vi "AO SCTR Engine.vi"(0 "Unique Notifier Name":string, 11 "AO PFI Lines":string[](array[string])) -> ()   [LabVIEW 2016]
uses:
  AO SCTR Type Defs/AO SCTR Notifier Type.ctl
  AO SCTR Type Defs/AO SCTR Actions.ctl
  <vilib>/DAQmx/write.llb/DAQmx Write (Analog DBL 1Chan 1Samp).vi
  <vilib>/Analysis/1siggen.llb/Ramp Pattern by Samples.vi
  <vilib>/DAQmx/write.llb/DAQmx Write (Analog 1D DBL 1Chan NSamp).vi
  <vilib>/DAQmx/create/channels.llb/DAQmx Create Channel (AO-Voltage-Basic).vi
  <vilib>/DAQmx/miscellaneous.llb/DAQmx Fill In Error Info.vi
  <vilib>/DAQmx/configure/timing.llb/DAQmx Timing (Sample Clock).vi
  <resource>/objmgr/daqmx.rc
  <vilib>/Analysis/NI_AALBase.lvlib
panel:
  out "Running":bool
  in  "Load":bool
  in  "Save":bool
  in  "Quit":bool
  in  "Waveform Settings":T1={"Actions"=enum."Offset", "Mirror Offset (V)"=-0.61, "Mirror Amplititude (V)"=0.524, "Samples Per Channel"=2280, "Start Delay (ms)"=20.0, "Running?"=FALSE} {"Mirror Amplititude (V)" format="%#_13g"; "Mirror Offset (V)" format="%#_13g"; "Start Delay (ms)" format="%#_13g"}
  out "Waveform Graph":dbl[](graph)
  out "Actual Sample Rate":dbl=10000.0 format="%0.2f"
  # "AO Line Example: Dev1/ao1\nPFI Line Example: /Dev1/PFI0"
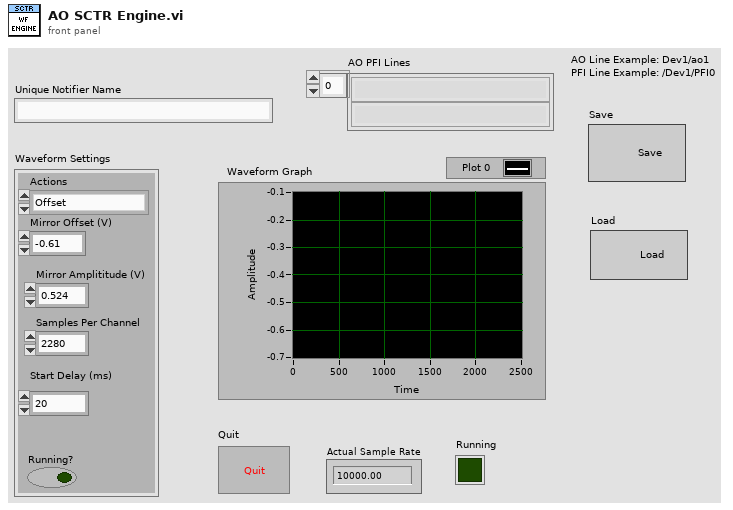
[diagram p1: front panel]
types:
  T1 = typedef "AO SCTR Notifier Type.ctl" = cluster{"Actions":T2, "Mirror Offset (V)":dbl, "Mirror Amplititude (V)":dbl, "Samples Per Channel":i32, "Start Delay (ms)":dbl, "Running?":bool}
  T2 = typedef "AO SCTR Actions.ctl" = enum16{"Offset", "Run", "Quit"}
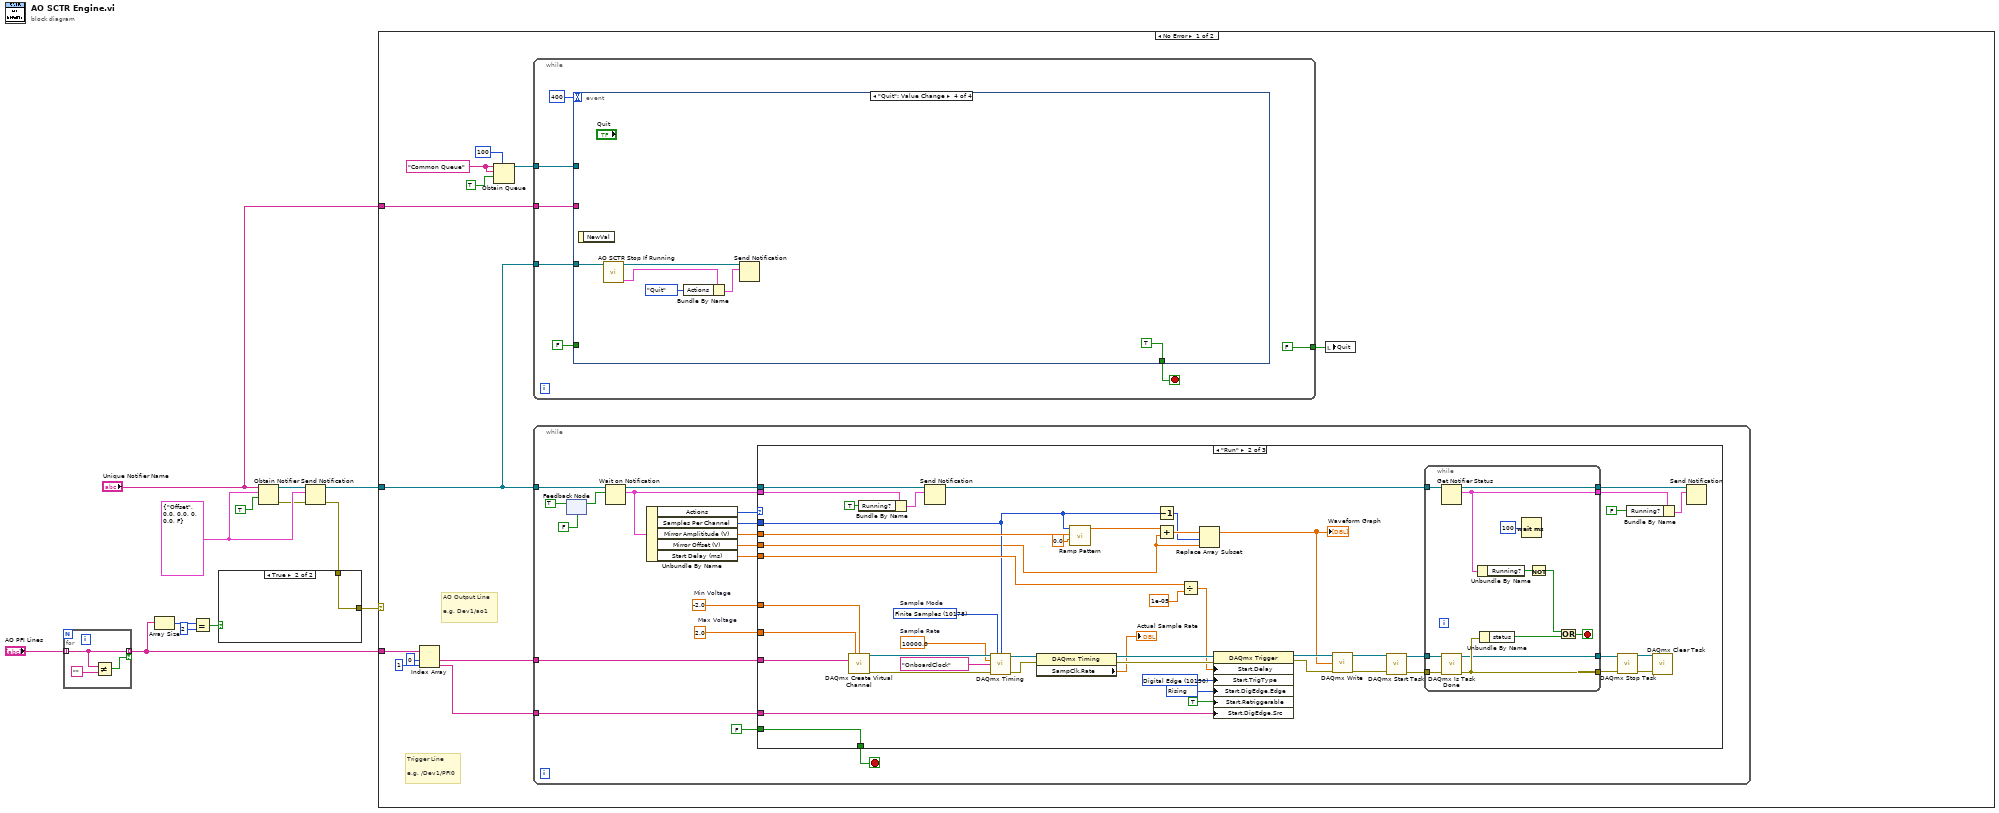
[diagram p0: block diagram]
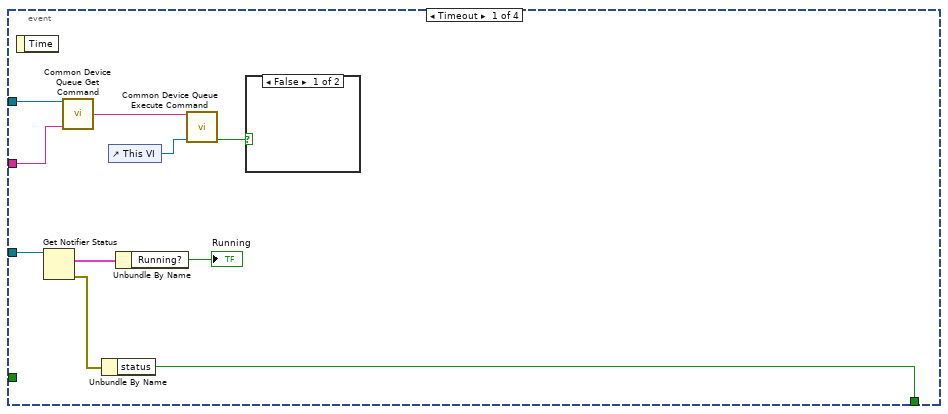
[diagram p2: hidden frame]
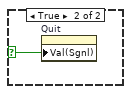
[diagram p3: hidden frame]
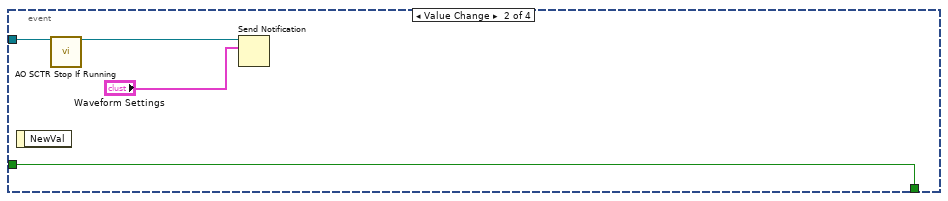
[diagram p4: hidden frame]
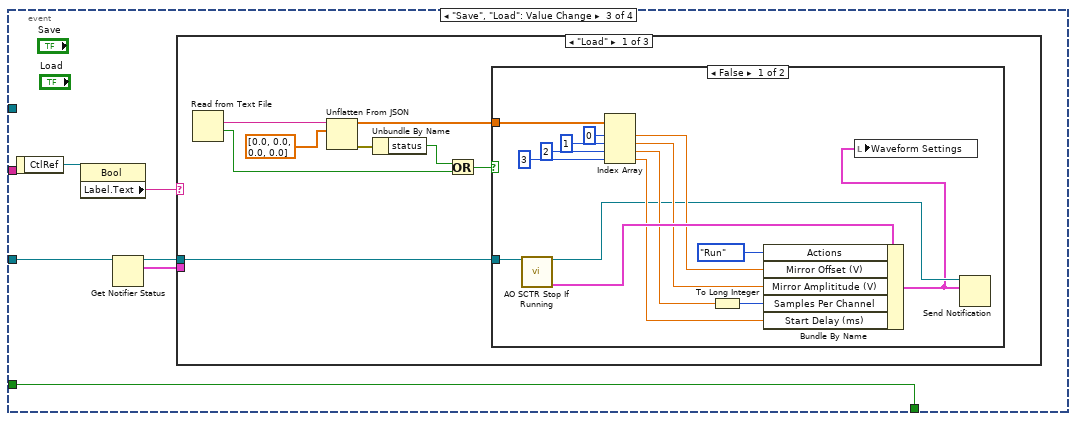
[diagram p5: hidden frame]
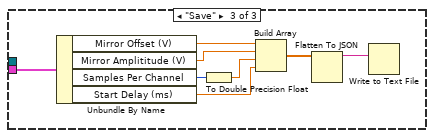
[diagram p8: hidden frame]
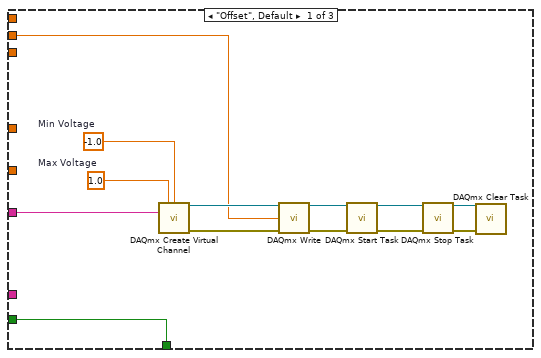
[diagram p9: hidden frame]
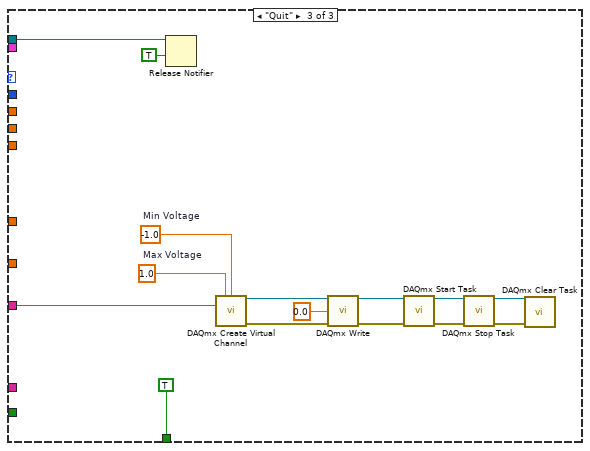
[diagram p10: hidden frame]
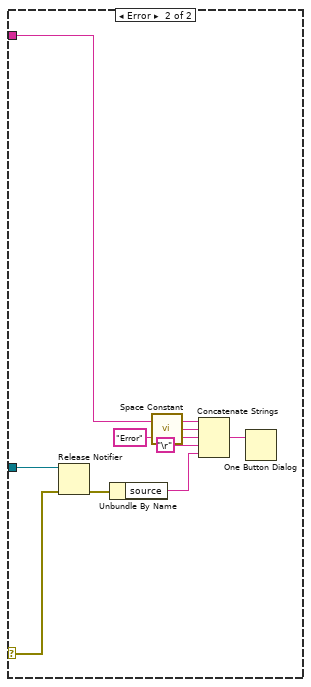
[diagram p11: hidden frame]
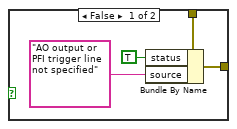
[diagram p12: hidden frame]
diagram:
  w8 = T1 {"Actions"=enum."Offset", "Mirror Offset (V)"=0.0, "Mirror Amplititude (V)"=0.0, "Samples Per Channel"=0, "Start Delay (ms)"=0.0, "Running?"=FALSE} ("Waveform Settings 2")
  n1 = for {
    tunnel: "AO PFI Lines" -> [w15] mode=indexing
    tunnel: [w15] -> w6 mode=indexing if=w14
    n2 = Not Equal?(x=w15, y="") -> (x != y?=w14:bool)
  }
  n3 = Array Size(array=w6) -> (size(s)=w5:i32)
  n4 = Equal?(x=w5, y=2) -> (x = y?=w3:bool)
  n5 = Obtain Notifier(name (unnamed)="Unique Notifier Name", notification data type=w8, create if not found? (T)=TRUE) -> (notifier out=w10:refnum<notifier>, error out=w7:errorcluster)  [unwired: 1 in, 1 out]
  n6 = Send Notification(notification=w8, notifier=w10, error in (no error)=w7) -> (notifier out=w9:refnum<notifier>, error out=w2:errorcluster)
  n7 = case shown="True" w3 {
    tunnel: w2 -> [w20 w21]
    tunnel: [w19 w21] -> w1
    frame False {
      n8 = Bundle By Name(cluster=w20, "status"=TRUE, "source"="AO output or PFI trigger line not specified") -> (w19:errorcluster)
    }
    frame True {
    }
  }
  n9 = case shown="No Error" w1 {
    selector: w1 -> [_ w211]
    tunnel: "Unique Notifier Name" -> [w28 w209]
    tunnel: w9 -> [w23 w212]
    tunnel: w6 -> [w22 _]
    frame No Error {
      w33 = "Common Queue" ("Unique Notifier Name")
      # "Trigger Line\n\ne.g. /Dev1/PFI0"
      # "AO Output Line\n\ne.g. Dev1/ao1"
      n10 = Index Array(array=w22, index #1=0 ("index"), index #2=1 ("index")) -> (element #1=w25:string, element #2=w24:string)
      n11 = Obtain Queue(max queue size (-1, unlimited)=100, name (unnamed)=w33, element data type=w33, create if not found? (T)=TRUE) -> (queue out=w29:refnum<queue>)  [unwired: 1 in, 2 out]
      n12 = while {
        tunnel: w23 -> [w40]
        tunnel: [FALSE] -> w30
        tunnel: w29 -> [w36]
        tunnel: w28 -> [w35]
        stop <- w38 stop-if-true
        n13 = event shown="[3] \"Quit\": Value Change" {
          selector: _ -> [_ _ _ _]
          dyn-events: _ -> [_ _ _ _]
          timeout: 400 -> [_ _ _ _]
          tunnel: w40 -> [w50 w53 w59 w95]
          tunnel: [w48 w55 w56 TRUE ("status")] -> w38
          tunnel: w36 -> [w44 _ _ _]
          tunnel: w35 -> [w43 _ _ _]
          tunnel: FALSE ("status") -> [_ w55 w56 _]
          event Timeout {
            n14 = event-data() -> ()  [unwired: 1 in, 1 out]
            n15 = Get Notifier Status(notifier=w50) -> (current notification=w42:T1, error out=w49:errorcluster)  [unwired: 1 in, 3 out]
            n16 = call "Common Device Queue Get Command.vi"("Common Queue"=w44, "Notifier Name"=w43) -> ("Command"=w46:string)  [unwired: 12 in, 1 out]
            n17 = Unbundle By Name(w49) -> ("status"=w48:bool)
            n18 = control-ref of="This VI"() -> (w45:refnum<vi>)
            n19 = Unbundle By Name(w42) -> ("Running?"=→"Running":bool)
            n20 = call "Common Device Queue Execute Command.vi"("Common Command"=w46, "VI Refnum"=w45) -> ("Quit?"=w47:bool)  [unwired: 12 in, 1 out]
            n21 = case shown="False" w47 {
              selector: w47 -> [_ w51]
              frame False {
              }
              frame True {
                n22 = property on="Quit" class="Bool (strict)"("Val(Sgnl)"=w51) -> ()  [unwired: 2 in, 2 out]
              }
            }
          }
          event Value Change {
            n23 = event-data() -> ()  [unwired: 1 in, 1 out]
            n24 = call "AO SCTR Stop If Running.vi"("AO SCTR Notifier"=w53) -> ("AO SCTR Notifier (Dup)"=w52:refnum<notifier>)  [unwired: 13 in, 1 out]
            n25 = Send Notification(notification="Waveform Settings", notifier=w52) -> ()  [unwired: 1 in, 2 out]
          }
          event "Save", "Load": Value Change {
            n26 = event-data() -> ("CtlRef"=w61:refnum<vi>)  [unwired: 1 in]
            n27 = property class="Bool"(reference=w61) -> ("Label.Text"=w60:string)  [unwired: 1 in, 2 out]
            n28 = Get Notifier Status(notifier=w59) -> (notifier out=w57:refnum<notifier>, current notification=w58:T1)  [unwired: 1 in, 3 out]
            n29 = case shown="\"Load\"" w60 {
              tunnel: w58 -> [_ _ w92]
              tunnel: w57 -> [w63 _ _]
              frame "Load" {
                n30 = Read from Text File() -> (text=w69:string, cancelled=w65:bool)  [unwired: 4 in, 2 out]
                n31 = Unflatten From JSON(JSON string=w69, type and defaults=dbl[] [0.0, 0.0, 0.0, 0.0]) -> (value=w62:dbl[], error out=w67:errorcluster)  [unwired: 5 in]
                n32 = Unbundle By Name(w67) -> ("status"=w66:bool)
                n33 = Or(x=w66, y=w65) -> (x .or. y?=w64:bool)
                n34 = case shown="False" w64 {
                  tunnel: w63 -> [w84 _]
                  tunnel: w62 -> [w81 _]
                  frame False {
                    n35 = call "AO SCTR Stop If Running.vi"("AO SCTR Notifier"=w84) -> ("AO SCTR Notifier (Dup)"=w71:refnum<notifier>, "Latest Notification"=w83:T1)  [unwired: 13 in]
                    n36 = Index Array(array=w81, index #1=0 ("index"), index #2=1 ("index"), index #3=2 ("index"), index #4=3 ("index")) -> (element #1=w72:dbl, element #2=w73:dbl, element #3=w75:dbl, element #4=w76:dbl)
                    n37 = To Long Integer(number=w75) -> (32bit integer=w74:i32)
                    n38 = Bundle By Name(cluster=w83, "Actions"=AO_SCTR_Actions."Run", "Mirror Offset (V)"=w72, "Mirror Amplititude (V)"=w73, "Samples Per Channel"=w74, "Start Delay (ms)"=w76) -> (w70:T1)
                    n39 = local write "Waveform Settings"(w70) -> ()
                    n40 = Send Notification(notification=w70, notifier=w71) -> ()  [unwired: 1 in, 2 out]
                  }
                  frame True {
                  }
                }
              }
              frame Default {
              }
              frame "Save" {
                n41 = Unbundle By Name(w92) -> ("Mirror Offset (V)"=w91:dbl, "Mirror Amplititude (V)"=w88:dbl, "Samples Per Channel"=w89:i32, "Start Delay (ms)"=w90:dbl)
                n42 = To Double Precision Float(number=w89) -> (double precision float=w87:dbl)
                n43 = Build Array(w91, w88, w87, w90) -> (w86:dbl[])
                n44 = Flatten To JSON(anything=w86) -> (JSON string=w85:string)  [unwired: 2 in, 1 out]
                n45 = Write to Text File(text=w85) -> ()  [unwired: 3 in, 3 out]
              }
            }
          }
          event "Quit": Value Change {
            n46 = event-data() -> ()  [unwired: 1 in, 1 out]
            n47 = call "AO SCTR Stop If Running.vi"("AO SCTR Notifier"=w95) -> ("AO SCTR Notifier (Dup)"=w94:refnum<notifier>, "Latest Notification"=w93:T1)  [unwired: 13 in]
            n48 = Bundle By Name(cluster=w93, "Actions"=AO_SCTR_Actions."Quit") -> (w97:T1)
            n49 = Send Notification(notification=w97, notifier=w94) -> ()  [unwired: 1 in, 2 out]
          }
        }
      }
      n50 = while {
        tunnel: w23 -> [w99]
        tunnel: w25 -> [w107]
        tunnel: w24 -> [w106]
        stop <- w108 stop-if-true
        w101 = 2.0  # Max Voltage
        w102 = -2.0  # Min Voltage
        n51 = feedback-in #1(TRUE ("ignore previous (F)")) -> ()
        n52 = feedback #1(FALSE ("ignore previous (F)")) -> (w103:bool)
        n53 = Wait on Notification(notifier=w99, ignore previous (F)=w103) -> (notifier out=w110:refnum<notifier>, notification=w109:T1)  [unwired: 2 in, 2 out]
        n54 = Unbundle By Name(w109) -> ("Actions"=w111:T2, "Samples Per Channel"=w113:i32, "Mirror Amplititude (V)"=w115:dbl, "Mirror Offset (V)"=w112:dbl, "Start Delay (ms)"=w114:dbl)
        n55 = case shown="\"Run\"" w111 {
          tunnel: w115 -> [_ w146 _]
          tunnel: w114 -> [_ w145 _]
          tunnel: w113 -> [_ w144 _]
          tunnel: w112 -> [w118 w143 _]
          tunnel: w110 -> [_ w142 w201]
          tunnel: w109 -> [_ w140 _]
          tunnel: [w117 w134 TRUE] -> w108
          tunnel: w107 -> [w116 w137 w189]
          tunnel: w106 -> [_ w129 _]
          tunnel: w102 -> [_ w136 _]
          tunnel: w101 -> [_ w135 _]
          tunnel: FALSE -> [w117 w134 _]
          frame "Offset", Default {
            w120 = 1.0  # Max Voltage
            w119 = -1.0  # Min Voltage
            n56 = call-poly <vilib>:"DAQmx Create Virtual Channel.vi"("maximum value"=w120, "minimum value"=w119, "physical channels"=w116) -> ("task out"=w121:refnum<k21>, "error out"=w126:errorcluster)  [unwired: 11 in]
            n57 = call-poly <vilib>:"DAQmx Write.vi"("task/channels in"=w121, "data"=w118, "error in"=w126) -> ("task out"=w122:refnum<k21>, "error out"=w127:errorcluster)  [unwired: 10 in, 1 out]
            n58 = call <vilib>:"DAQmx Start Task.vi"("task/channels in"=w122, "error in"=w127) -> ("task out"=w124:refnum<k21>, "error out"=w128:errorcluster)  [unwired: 12 in]
            n59 = call <vilib>:"DAQmx Stop Task.vi"("task/channels in"=w124, "error in"=w128) -> ("task out"=w125:refnum<k21>, "error out"=w123:errorcluster)  [unwired: 12 in]
            n60 = call <vilib>:"DAQmx Clear Task.vi"("task in"=w125, "error in"=w123) -> ()  [unwired: 13 in, 1 out]
          }
          frame "Run" {
            w169 = 10000.0  # Sample Rate
            w159 = 10280 items=["Rising"=10280, "Falling"=10171] ("Start.DigEdge.Edge")
            w148 = 10150 items=["Analog Edge"=10099, "Digital Edge"=10150, "Digital Pattern"=10398, "Analog Window"=10103, "None"=10230] ("Start.TrigType")
            w175 = 10178 items=["Finite Samples"=10178, "Continuous Samples"=10123, "Hardware Timed Single Point"=12522]  # Sample Mode
            n61 = call-poly <vilib>:"DAQmx Create Virtual Channel.vi"("maximum value"=w135, "minimum value"=w136, "physical channels"=w137) -> ("task out"=w173:refnum<k21>, "error out"=w174:errorcluster)  [unwired: 11 in]
            n62 = Bundle By Name(cluster=w140, "Running?"=TRUE ("Running")) -> (w138:T1)
            n63 = Send Notification(notification=w138, notifier=w142) -> (notifier out=w141:refnum<notifier>)  [unwired: 1 in, 1 out]
            n64 = call-poly <vilib>:"DAQmx Timing.vi"("task/channels in"=w173, "sample mode"=w175, "samples per channel"=w144, "rate"=w169, "source"=tag "OnboardClock" ("Sample Clock Source"), "error in"=w174) -> ("task out"=w157:refnum<k21>, "error out"=w176:errorcluster)  [unwired: 8 in]
            n65 = property class="DAQmx Timing"(reference=w157, error in=w176) -> (reference out=w162:refnum<k21>, error out=w161:errorcluster, "SampClk.Rate"=→"Actual Sample Rate":dbl)
            n66 = call-poly <vilib>:"Ramp Pattern.vi"("start"=0.0, "end"=w146, "samples"=w144) -> ("Ramp Pattern"=w153:dbl[])  [unwired: 7 in, 1 out]
            n67 = Decrement(x=w144) -> (x-1=w151:i32)
            n68 = Add(x=w153, y=w143) -> (x+y=w152:dbl[])
            n69 = Divide(x=w145, y=1e-05) -> (x/y=w147:dbl)
            n70 = Replace Array Subset(array=w152, new element=w143, index=w151) -> (w150:dbl[])
            "Waveform Graph" <- w150
            n71 = property class="DAQmx Trigger"(reference=w162, error in=w161, "Start.Delay"=w147, "Start.TrigType"=w148, "Start.DigEdge.Edge"=w159, "Start.Retriggerable"=TRUE, "Start.DigEdge.Src"=w129) -> (reference out=w160:refnum<k21>, error out=w154:errorcluster)
            n72 = call-poly <vilib>:"DAQmx Write.vi"("task/channels in"=w160, "data"=w150, "error in"=w154) -> ("task out"=w168:refnum<k21>, "error out"=w167:errorcluster)  [unwired: 10 in, 1 out]
            n73 = call <vilib>:"DAQmx Start Task.vi"("task/channels in"=w168, "error in"=w167) -> ("task out"=w172:refnum<k21>, "error out"=w171:errorcluster)  [unwired: 12 in]
            n74 = while {
              tunnel: w172 -> [w188]
              tunnel: w171 -> [w187]
              tunnel: [w186] -> w163
              tunnel: [w185] -> w164
              tunnel: w141 -> [w182]
              tunnel: [w180] -> w133
              tunnel: [w179] -> w130
              stop <- w184 stop-if-true
              n75 = Get Notifier Status(notifier=w182) -> (notifier out=w180:refnum<notifier>, current notification=w179:T1)  [unwired: 1 in, 3 out]
              n76 = call <vilib>:"DAQmx Is Task Done.vi"("task/channels in"=w188, "error in"=w187) -> ("task out"=w185:refnum<k21>, "error out"=w186:errorcluster)  [unwired: 11 in, 1 out]
              n77 = Unbundle By Name(w179) -> ("Running?"=w181:bool)
              n78 = Unbundle By Name(w186) -> ("status"=w183:bool)
              n79 = Wait (ms)(milliseconds to wait=u32 100) -> ()  [unwired: 1 out]
              n80 = Not(x=w181) -> (.not. x?=w178:bool)
              n81 = Or(x=w178, y=w183) -> (x .or. y?=w184:bool)
            }
            n82 = call <vilib>:"DAQmx Stop Task.vi"("task/channels in"=w164, "error in"=w163) -> ("task out"=w166:refnum<k21>, "error out"=w165:errorcluster)  [unwired: 12 in]
            n83 = Bundle By Name(cluster=w130, "Running?"=FALSE ("Running")) -> (w131:T1)
            n84 = call <vilib>:"DAQmx Clear Task.vi"("task in"=w166, "error in"=w165) -> ()  [unwired: 13 in, 1 out]
            n85 = Send Notification(notification=w131, notifier=w133) -> ()  [unwired: 1 in, 2 out]
          }
          frame "Quit" {
            w192 = 1.0  # Max Voltage
            w191 = -1.0  # Min Voltage
            n86 = Release Notifier(notifier=w201, force destroy? (F)=TRUE) -> ()  [unwired: 1 in, 3 out]
            n87 = call-poly <vilib>:"DAQmx Create Virtual Channel.vi"("maximum value"=w192, "minimum value"=w191, "physical channels"=w189) -> ("task out"=w193:refnum<k21>, "error out"=w198:errorcluster)  [unwired: 11 in]
            n88 = call-poly <vilib>:"DAQmx Write.vi"("task/channels in"=w193, "data"=0.0, "error in"=w198) -> ("task out"=w194:refnum<k21>, "error out"=w199:errorcluster)  [unwired: 10 in, 1 out]
            n89 = call <vilib>:"DAQmx Start Task.vi"("task/channels in"=w194, "error in"=w199) -> ("task out"=w196:refnum<k21>, "error out"=w200:errorcluster)  [unwired: 12 in]
            n90 = call <vilib>:"DAQmx Stop Task.vi"("task/channels in"=w196, "error in"=w200) -> ("task out"=w197:refnum<k21>, "error out"=w195:errorcluster)  [unwired: 12 in]
            n91 = call <vilib>:"DAQmx Clear Task.vi"("task in"=w197, "error in"=w195) -> ()  [unwired: 13 in, 1 out]
          }
        }
      }
      n92 = local write "Quit"(w30) -> ()
    }
    frame Error {
      n93 = Release Notifier(notifier=w212, error in (no error)=w211) -> (error out=w205:errorcluster)  [unwired: 1 in, 2 out]
      n94 = Unbundle By Name(w205) -> ("source"=w204:string)
      n95 = call <vilib>:"Space Constant.vi"() -> ("String"=w208:string)
      n96 = Concatenate Strings(w209, w208, "Error" ("string"), "\r", w204) -> (w210:string)
      n97 = One Button Dialog(message=w210) -> ()  [unwired: 1 in, 1 out]
    }
  }
